vi "Resource Library Path.vi"(11 "Relative Path":path) -> (3 "Resource + Relative Path":path)   [LabVIEW 2013, in "Scripter.lvlib"]
uses:
  Scripter.lvlib
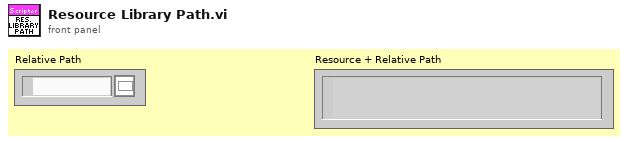
[diagram p1: front panel]
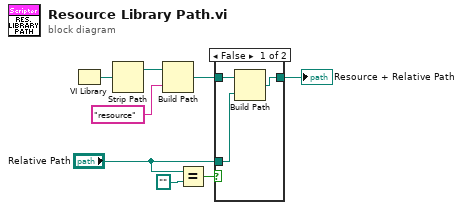
[diagram p0: block diagram]
diagram:
  n1 = VI Library() -> (path=w8:path)
  n2 = Strip Path(path=w8) -> (stripped path=w7:path)  [unwired: 1 out]
  n3 = Build Path(base path=w7, name or relative path="resource") -> (appended path=w5:path)
  n4 = Equal?(x="Relative Path", y=path "") -> (x = y?=w1:bool)
  n5 = case shown="False" w1 {
    tunnel: w5 -> [w11 w12]
    tunnel: [w10 w12] -> w4
    tunnel: "Relative Path" -> [w9 _]
    frame False {
      n6 = Build Path(base path=w11, name or relative path=w9) -> (appended path=w10:path)
    }
    frame True {
    }
  }
  "Resource + Relative Path" <- w4
